vi "sym matrix to compact form.vi"(10 "Preallocated Compact Form":dbl[](array[numeric]), 11 "Symmetric Matrix":T1) -> (2 "Compact Form":dbl[](array[numeric]))   [LabVIEW 2010, in "NI_AALPro.lvlib"]
uses:
  NI_AALPro.lvlib
  RealMatrix.ctl
  lvanlys.dll
  NI_Matrix.lvlib
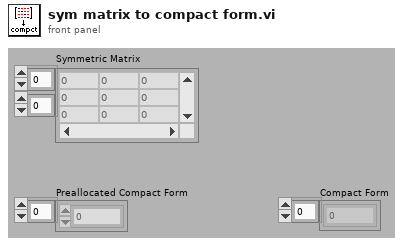
[diagram p1: front panel]
types:
  T1 = typedef "NI_Matrix.lvlib/RealMatrix.ctl" = dbl[][]
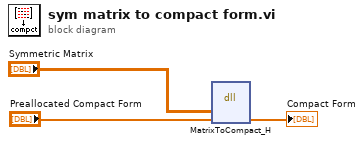
[diagram p0: block diagram]
diagram:
  n1 = dll-call lib="C:/Program Files/National Instruments/LabVIEW 2010/resource/lvanlys.*" fn="MatrixToCompact_H"("matrixH"="Symmetric Matrix", "aH"="Preallocated Compact Form") -> ("aH"=→"Compact Form":dbl[])  [unwired: 5 in, 2 out]
